vi "Launch Serial Actor.vi"(8 "error in":errorcluster, 11 "PS in":refnum<class "Power Supply.lvclass">) -> (0 "error out":errorcluster, 3 "PS out":refnum<class "Power Supply.lvclass">)   [LabVIEW 2019, in "Power Supply.lvlib" / "Power Supply.lvclass"]
uses:
  Power Supply.lvclass
  C:/Program Files (x86)/National Instruments/LabVIEW 2019/vi.lib/ActorFramework/Actor/Actor.lvclass
  Serial/Serial/Serial.lvclass
  Power Supply Messages/Receive Response Msg/Receive Response Msg.lvclass
  C:/Working Copy/trunk/Modified Cobra Jung/Cobra/Cobra AF/Serial/Serial Messages/Response Msg/Response Msg.lvclass
  Serial/Serial/Serial.lvclass/Serial.ctl
  Power Supply.lvclass/Power Supply.ctl
  <vilib>/ActorFramework/Actor/Actor.lvclass
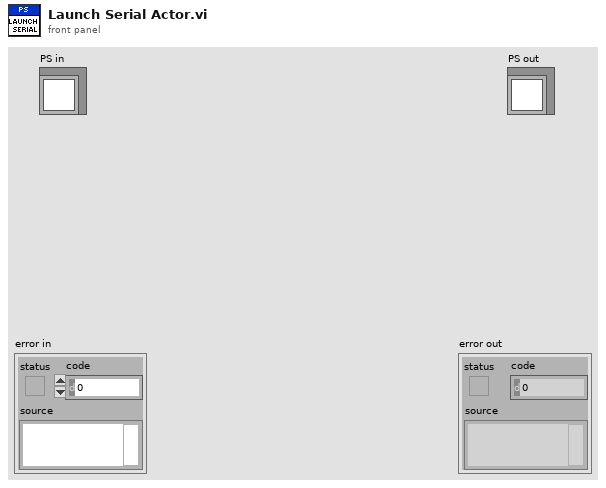
[diagram p1: front panel]
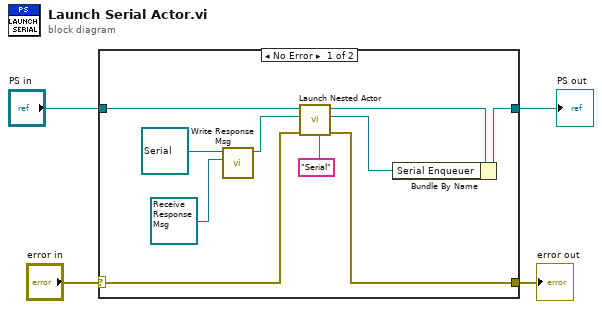
[diagram p0: block diagram]
diagram:
  n1 = case shown="No Error" "error in" {
    selector: "error in" -> [w11 w16]
    tunnel: [w14 w16] -> w3
    tunnel: [w13 w15] -> w2
    tunnel: "PS in" -> [w12 w15]
    frame No Error {
      n2 = call "Write Response Msg.vi"("Serial.lvlib:Response Msg.lvclass"=refnum<class "Receive Response Msg.lvclass"> refnum ("Power Supply.lvlib:Receive Response Msg.lvclass"), "Serial in"=refnum<class "Serial.lvclass"> refnum ("Serial.lvlib:Serial.lvclass")) -> ("Serial out"=w7:refnum<class "Serial.lvclass">)  [unwired: 9 in]
      n3 = call <vilib>:"Launch Nested Actor.vi"("Debug Alias"="Serial", "error in (no error)"=w11, "Nested Actor"=w7, "Caller Actor in"=w12) -> ("error out"=w14:errorcluster, "Nested Actor's Enqueuer"=w6:refnum<class "Message Enqueuer.lvclass">, "Caller Actor out"=w9:refnum<class "Power Supply.lvclass">)  [unwired: 5 in]
      n4 = Bundle By Name(cluster=w9, "Serial Enqueuer"=w6) -> (w13:refnum<class "Power Supply.lvclass">)
    }
    frame Error {
    }
  }
  "error out" <- w3
  "PS out" <- w2
